vi "Test TDMS Read Speed.vi"(8 "error in (no error)":errorcluster, 11 "Path":path) -> (0 "error out":errorcluster, 2 "time (ms/file)":u32, 3 "dup Folder Path":path)   [LabVIEW 2016]
uses:
  LV to ITX/LV to ITX.lvclass
panel:
  in  "stop":bool
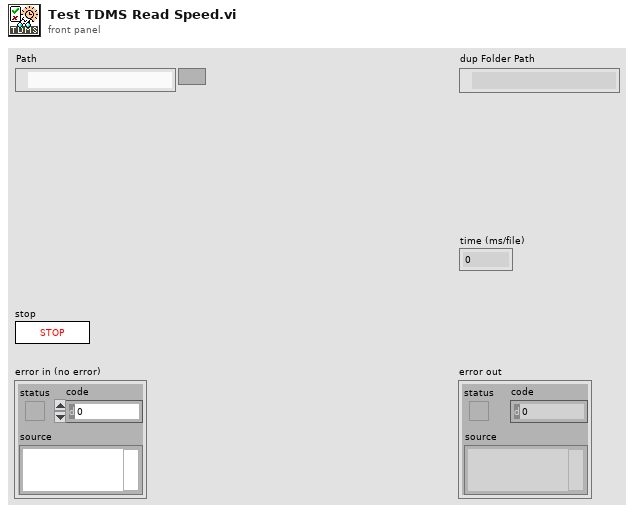
[diagram p1: front panel]
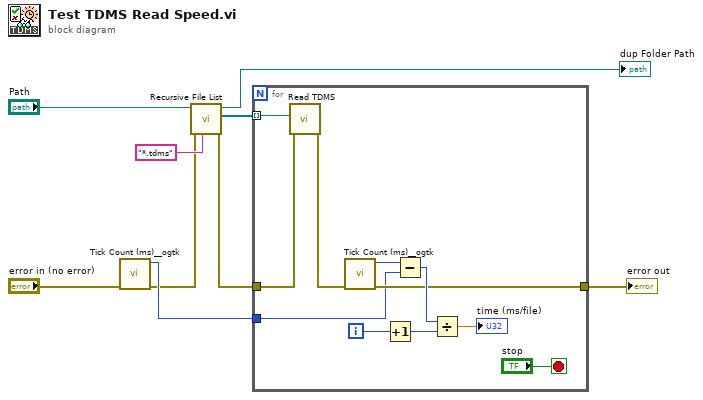
[diagram p0: block diagram]
diagram:
  n1 = call <userlib>:"Tick Count (ms)__ogtk.vi"("error in (no error)"="error in (no error)") -> ("error out"=w3:errorcluster, "millisecond timer value"=w5:u32)  [unwired: 9 in]
  n2 = call <vilib>:"Recursive File List.vi"("pattern"="*.tdms", "error in (no error)"=w3, "Folder Path"="Path") -> ("error out"=w2:errorcluster, "All Files in Dir"=w6:path[], "dup Folder Path"=→"dup Folder Path":path)  [unwired: 4 in, 2 out]
  n3 = for {
    tunnel: w6 -> [w20] mode=indexing
    tunnel: w2 -> [w12]
    tunnel: [w11] -> w4
    tunnel: w5 -> [w10]
    i -> [w18]
    stop <- "stop" stop-if-true
    n4 = call "Read TDMS.vi"("error in (no error)"=w12, "path"=w20) -> ("error out"=w16:errorcluster)  [unwired: 3 in, 6 out]
    n5 = call <userlib>:"Tick Count (ms)__ogtk.vi"("error in (no error)"=w16) -> ("error out"=w11:errorcluster, "millisecond timer value"=w13:u32)  [unwired: 9 in]
    n6 = Increment(x=w18) -> (x+1=w17:i32)
    n7 = Subtract(x=w13, y=w10) -> (x-y=w19:u32)
    n8 = Divide(x=w19, y=w17) -> (x/y=→"time (ms/file)":dbl)
  }
  "error out" <- w4
